vi "FTW-JSON-LexicalScan-FloatDeserialize.vi"(0 "Significant Digits":u8, 2 "Format":string, 7 "Byte Array":u8[](array[numeric])) -> (8 "Variant":variant)   [LabVIEW 2015]
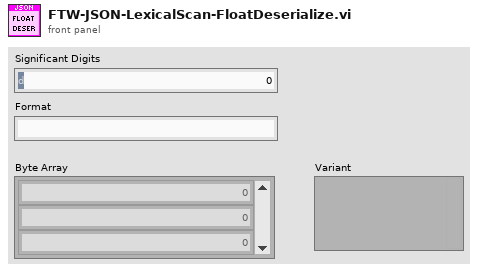
[diagram p1: front panel]
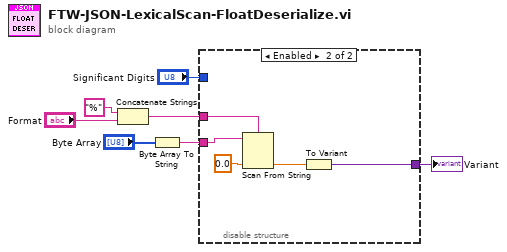
[diagram p0: block diagram]
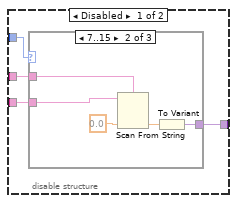
[diagram p2: hidden frame]
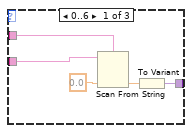
[diagram p3: hidden frame]
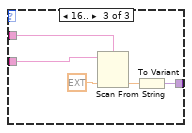
[diagram p4: hidden frame]
diagram:
  n1 = Concatenate Strings("%" ("string"), "Format") -> (w2:string)
  n2 = Byte Array To String(unsigned byte array="Byte Array") -> (string=w6:string)
  n3 = disable-structure shown="Enabled" {
    disable-tunnel: [w11 w27] -> w7
    disable-tunnel: w6 -> [w10 w28]
    disable-tunnel: "Significant Digits" -> [w9 _]
    disable-tunnel: w2 -> [w8 w29]
    frame Disabled {
      n4 = case shown="7..15" w9 {
        tunnel: [w16 w21 w26] -> w11
        tunnel: w10 -> [w13 w18 w23]
        tunnel: w8 -> [w12 w17 w22]
        frame 0..6 {
          n5 = Scan From String(format string=w12, input string=w13, default 1=sgl 0.0) -> (output 1=w15:sgl)  [unwired: 2 in, 3 out]
          n6 = To Variant(anything=w15) -> (Variant=w16:variant)
        }
        frame 7..15 {
          n7 = Scan From String(format string=w17, input string=w18, default 1=0.0) -> (output 1=w20:dbl)  [unwired: 2 in, 3 out]
          n8 = To Variant(anything=w20) -> (Variant=w21:variant)
        }
        frame 16.. {
          n9 = Scan From String(format string=w22, input string=w23, default 1=ext 0.0) -> (output 1=w25:ext)  [unwired: 2 in, 3 out]
          n10 = To Variant(anything=w25) -> (Variant=w26:variant)
        }
      }
    }
    frame Enabled {
      n11 = Scan From String(format string=w29, input string=w28, default 1=0.0) -> (output 1=w31:dbl)  [unwired: 2 in, 3 out]
      n12 = To Variant(anything=w31) -> (Variant=w27:variant)
    }
  }
  "Variant" <- w7
